vi "TLB Native Dynamic Events ver 0.05b queue mode.vi"() -> ()   [LabVIEW 2018]
uses:
  Labview Training Phase 2/Enum Controls/States for Action Engine.ctl
  Type def/TLB event states.ctl
  Type def/TLB MHL States.ctl
  <vilib>/Studica/Studica Toolkit/NavX/NavX.lvlib
  <vilib>/Studica/Studica Toolkit/Background/I2C Channel.ctl
  <vilib>/myRIO/Common/Instrument Driver Framework/myRIO v1.0/AI/typedefs/AI Channels Enum.ctl
  <vilib>/myRIO/Common/Instrument Driver Framework/myRIO v1.0/AI/typedefs/AI Channels List.ctl
panel:
  out "Sharp IR Distance 2":dbl
  out "Sharp IR Distance":dbl
  out "YRPHfH":T1
  out "Displacement":T2
  out "LinearAcceleration":T3
  out "NavX Info Out":T5
  out "Distance":T6
  out "Speed":T7
  in  "xTargetSpeed":dbl
  in  "yTargetSpeed":dbl
  in  "wTargetSpeed":dbl
  out "Action Queues":string[](array[string])
  out "State logic":T8
  out "Action State":string
  in  "Task condition":bool
  in  "Combo Box":string(combo)
  in  "Stop Queue":bool
  in  "Start Task":bool
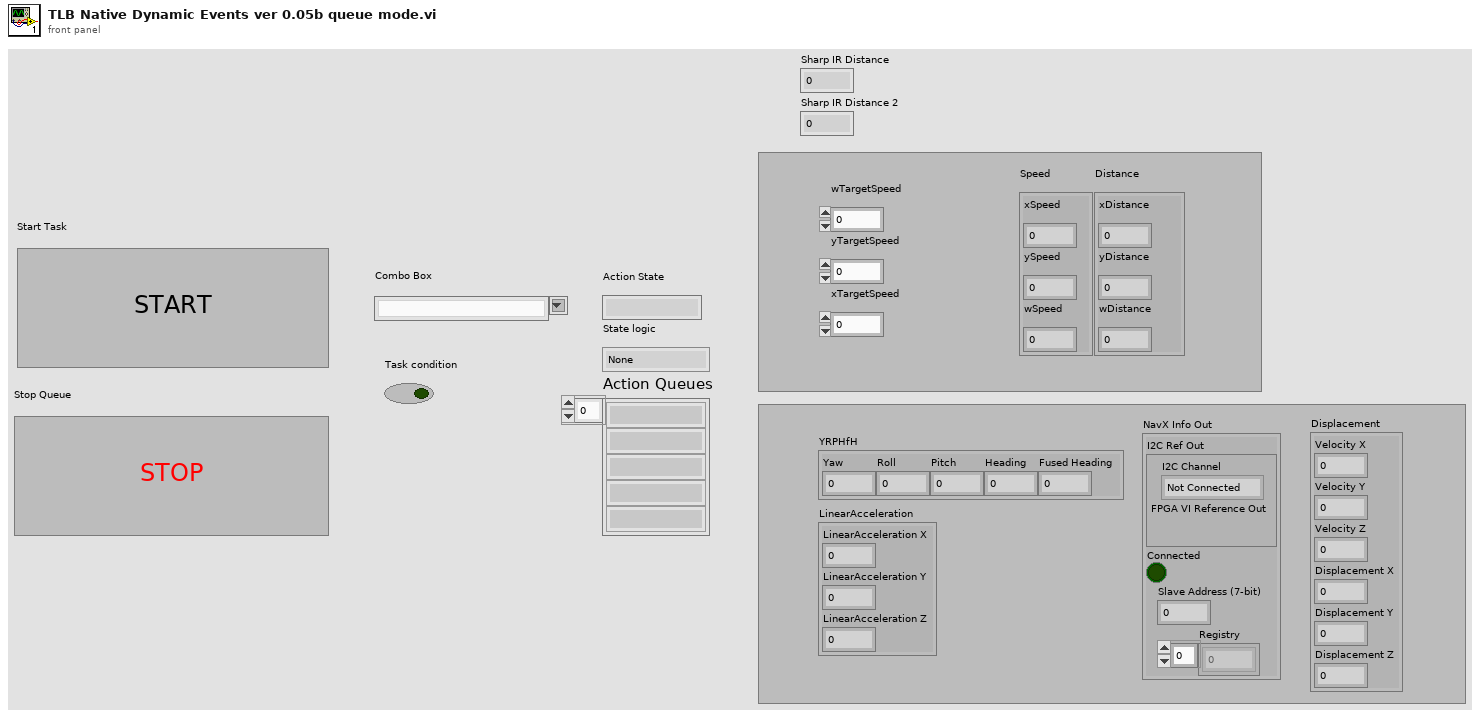
[diagram p1: front panel]
types:
  T1 = cluster{"Yaw":dbl, "Roll":dbl, "Pitch":dbl, "Heading":dbl, "Fused Heading":dbl}
  T2 = cluster{"Velocity X":dbl, "Velocity Y":dbl, "Velocity Z":dbl, "Displacement X":dbl, "Displacement Y":dbl, "Displacement Z":dbl}
  T3 = cluster{"LinearAcceleration X":dbl, "LinearAcceleration Y":dbl, "LinearAcceleration Z":dbl}
  T4 = typedef "I2C Channel.ctl" = enum16{"Not Connected", "A", "B"}
  T5 = cluster{"I2C Ref Out":cluster{"I2C Channel":T4, "FPGA VI Reference Out":refnum<k20>}, "Connected":bool, "Slave Address (7-bit)":u8, "Registry":u8[]}
  T6 = cluster{"xDistance":dbl, "yDistance":dbl, "wDistance":dbl}
  T7 = cluster{"xSpeed":dbl, "ySpeed":dbl, "wSpeed":dbl}
  T8 = typedef "TLB MHL States.ctl" = enum16{"None", "Startup", "Idle", "Processing", "Shutdown", "Reset", "Task 1", "Task 2", "Task 3", "Task 4", "Task 4a", "Task 4b", "Task 4c", "Task 4d", "Task 4e", "Task 4f", "Task 4g", "Task 4h", "Acquire image", "Wall follow mode", "Drive Straight"}
  T9 = typedef "States for Action Engine.ctl" = enum16{"Initialize", "Write", "Read"}
  T10 = typedef "TLB event states.ctl" = enum16{"Start Sequence", "Exit", "Start Task 1", "Start Task 2", "Start Task 3", "Start Task 4", "Camera vision", "Wall follow mode", "Idle", "Start Drive Straight"}
  T11 = typedef "TLB event states.ctl" = enum16{"Start Sequence", "Exit", "Task 1", "Task 2", "Idle"}
  T12 = cluster{"queue out":refnum<queue>, "error out":errorcluster}
  T13 = typedef "AI Channels List.ctl" = T14[]
  T14 = typedef "AI Channels Enum.ctl" = enum16{"Not Connected", "AudioIn/Left", "AudioIn/Right", "C/AI0", "C/AI1", "A/AI0", "A/AI1", "A/AI2", "A/AI3", "A/AI4", "A/AI5", "A/AI6", "A/AI7", "B/AI0", "B/AI1", "B/AI2", "B/AI3", "B/AI4", "B/AI5", "B/AI6", "B/AI7", "AI/AI0", "AI/AI1", "AI/AI2", "AI/AI3", "A/AI0 (DIFF)", "A/AI1 (DIFF)", "A/AI2 (DIFF)", "A/AI3 (DIFF)", "B/AI0 (DIFF)", "B/AI1 (DIFF)", "B/AI2 (DIFF)", "B/AI3 (DIFF)"}
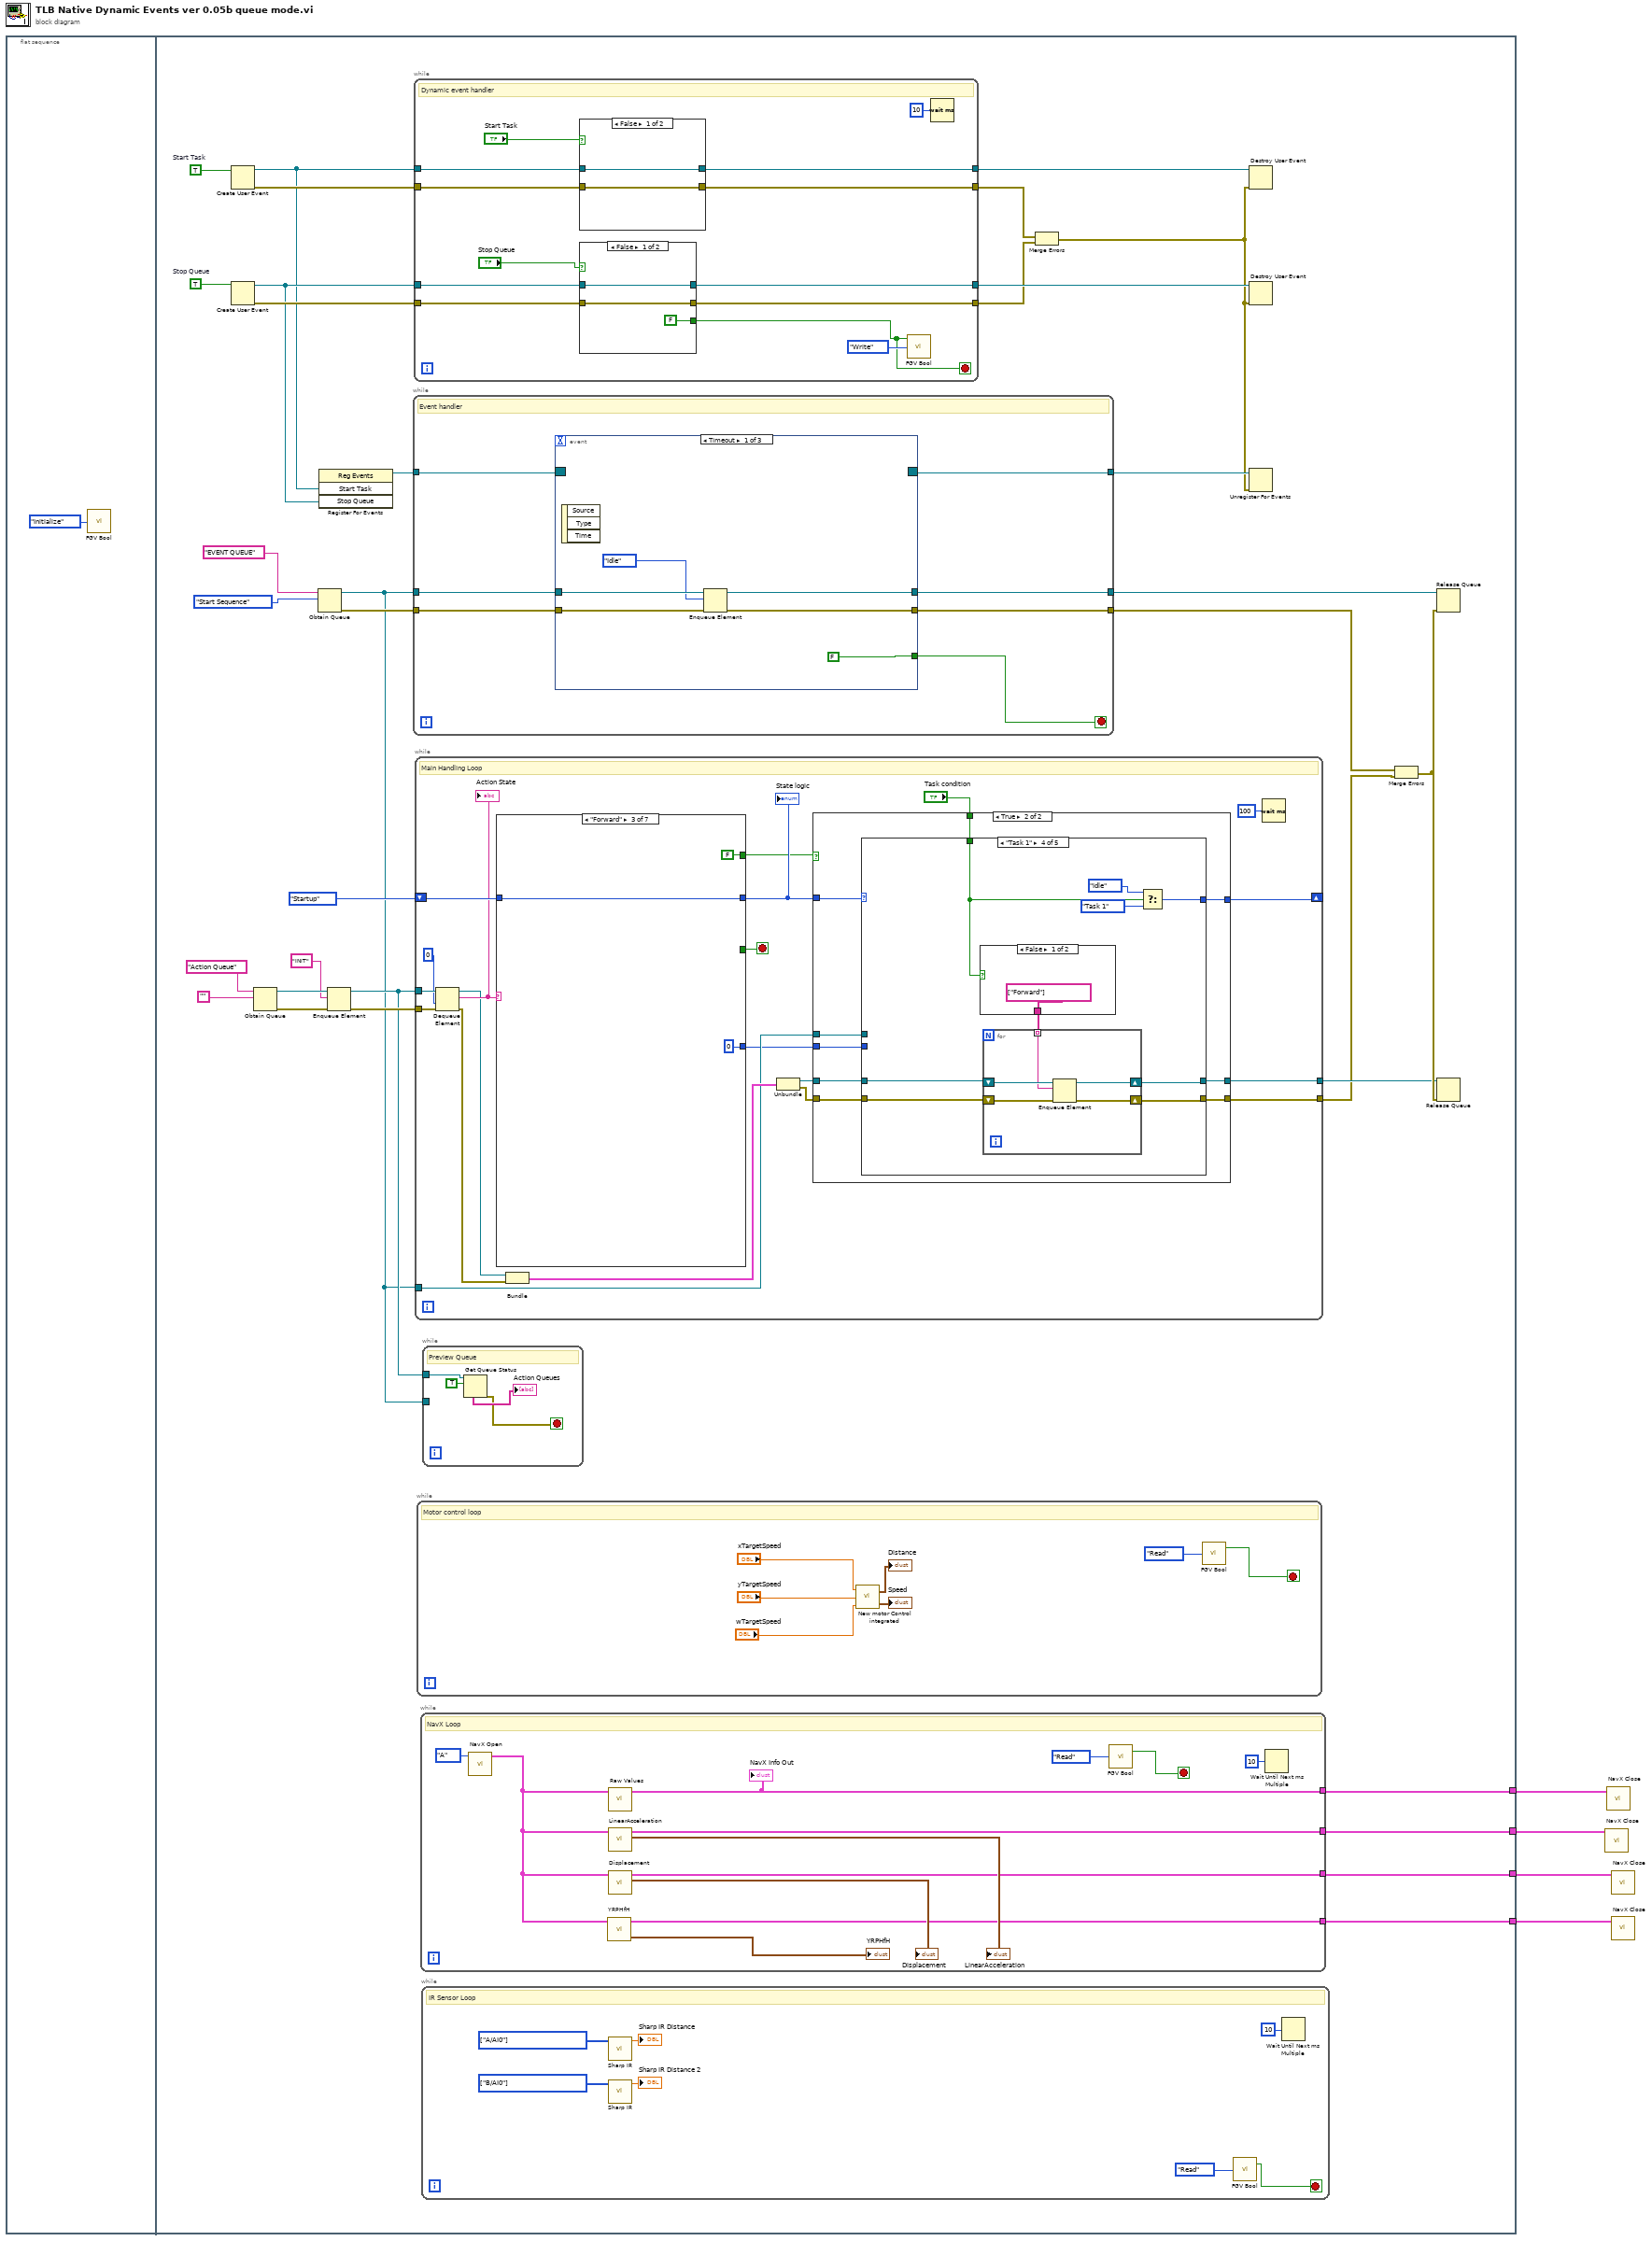
[diagram p0: block diagram]
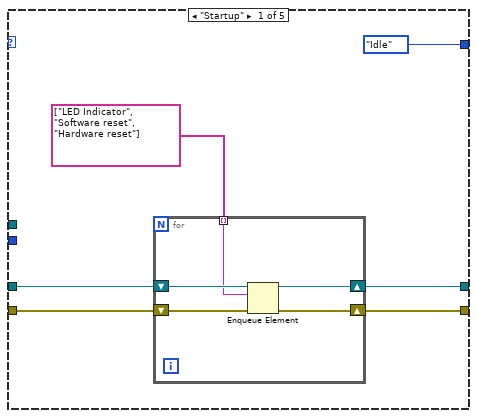
[diagram p3: hidden frame]
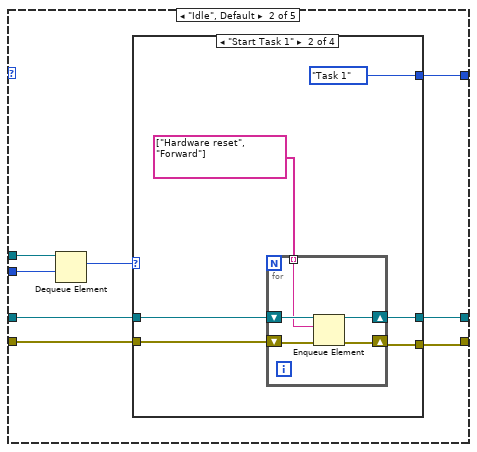
[diagram p4: hidden frame]
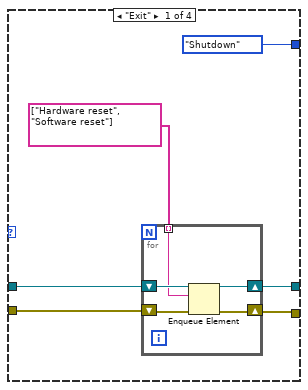
[diagram p5: hidden frame]
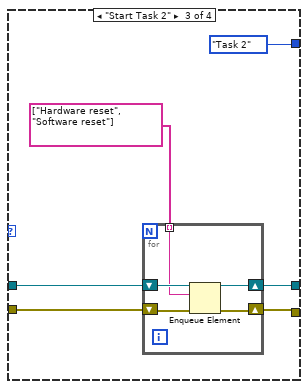
[diagram p6: hidden frame]
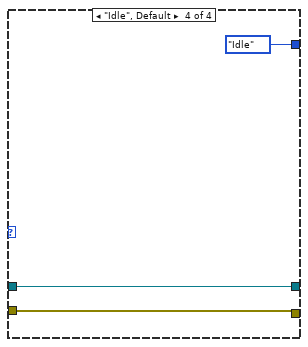
[diagram p7: hidden frame]
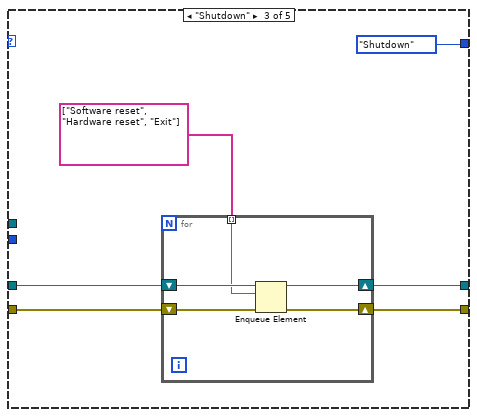
[diagram p8: hidden frame]
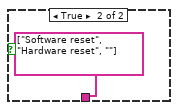
[diagram p9: hidden frame]
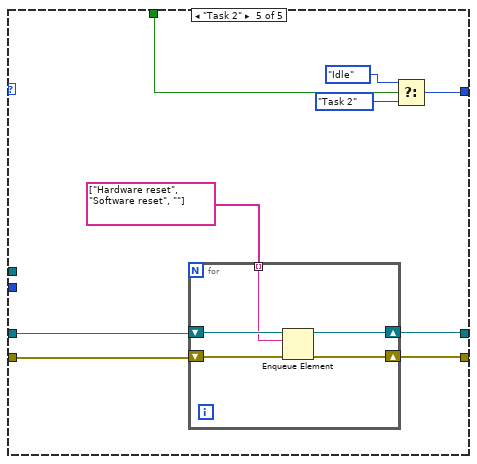
[diagram p10: hidden frame]
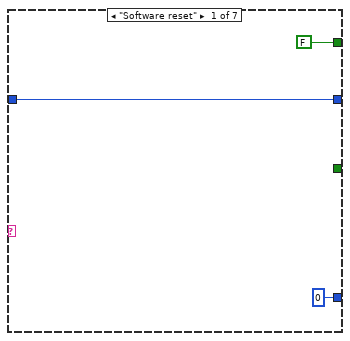
[diagram p11: hidden frame]
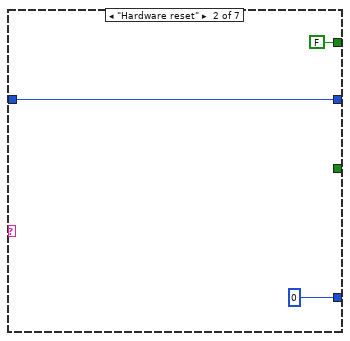
[diagram p12: hidden frame]
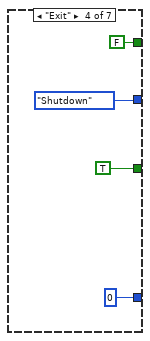
[diagram p13: hidden frame]
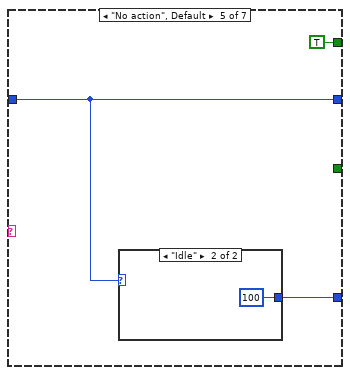
[diagram p14: hidden frame]
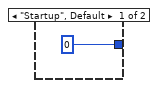
[diagram p15: hidden frame]
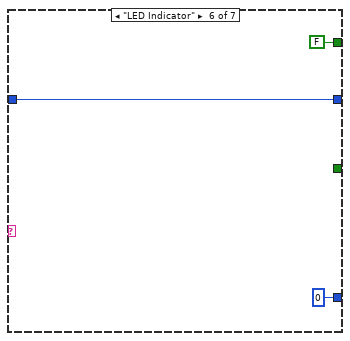
[diagram p16: hidden frame]
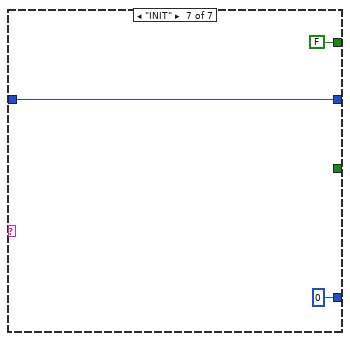
[diagram p17: hidden frame]
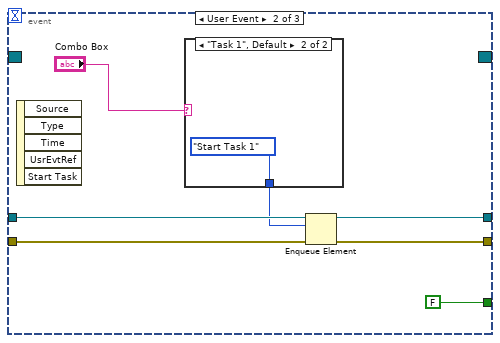
[diagram p18: hidden frame]
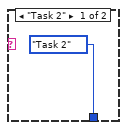
[diagram p19: hidden frame]
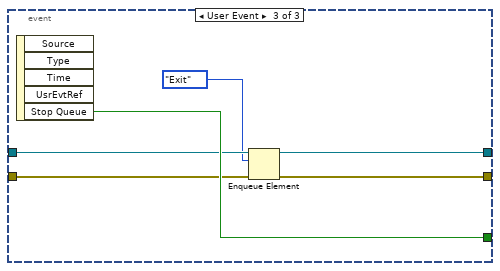
[diagram p20: hidden frame]
diagram:
  n1 = flat-sequence {
    tunnel: [w9] -> w4
    tunnel: [w8] -> w3
    tunnel: [w7] -> w2
    tunnel: [w6] -> w1
    frame #0 {
      n2 = call "FGV Bool.vi"("Init/Read/Write State"=States_for_Action_Engine."Initialize") -> ()  [unwired: 2 in, 2 out]
    }
    frame #1 {
      w39 = TRUE  # Stop Queue
      w38 = TRUE  # Start Task
      n3 = Create User Event(user event datatype=w38) -> (user event=w30:refnum<user-event>, error out=w35:errorcluster)  [unwired: 1 in]
      n4 = Create User Event(user event datatype=w39) -> (user event=w31:refnum<user-event>, error out=w34:errorcluster)  [unwired: 1 in]
      n5 = Obtain Queue(name (unnamed)="Action Queue", element data type="") -> (queue out=w23:refnum<queue>, error out=w19:errorcluster)  [unwired: 3 in, 1 out]
      n6 = Obtain Queue(name (unnamed)="EVENT QUEUE", element data type=TLB_event_states."Start Sequence" ("Enum")) -> (queue out=w10:refnum<queue>, error out=w20:errorcluster)  [unwired: 3 in, 1 out]
      n7 = register-events(w30, w31) -> (reference out=w29:refnum<event-registration>)  [unwired: 2 in, 1 out]
      n8 = Enqueue Element(queue=w23, element="INIT", error in (no error)=w19) -> (queue out=w11:refnum<queue>, error out=w18:errorcluster)  [unwired: 1 in, 1 out]
      n9 = while {
        tunnel: w29 -> [w228]
        tunnel: [w227] -> w28
        tunnel: w10 -> [w225]
        tunnel: [w224] -> w27
        tunnel: w20 -> [w223]
        tunnel: [w222] -> w17
        stop <- w226 stop-if-true
        # "Event handler"
        n10 = event shown="[0] Timeout" {
          selector: w228 -> [_ _ _]
          dyn-events: [_ _ _] -> w227
          timeout: _ -> [_ _ _]
          tunnel: [FALSE FALSE w249] -> w226
          tunnel: w225 -> [w233 w240 w247]
          tunnel: [w232 w239 w248] -> w224
          tunnel: w223 -> [w230 w236 w245]
          tunnel: [w229 w235 w244] -> w222
          event Timeout {
            n11 = event-data() -> ()  [unwired: 1 in, 3 out]
            n12 = Enqueue Element(queue=w233, element=TLB_event_states."Idle" ("Enum"), error in (no error)=w230) -> (queue out=w232:refnum<queue>, error out=w229:errorcluster)  [unwired: 1 in, 1 out]
          }
          event User Event {
            n13 = event-data() -> ()  [unwired: 1 in, 5 out]
            n14 = case shown="\"Task 1\", Default" "Combo Box" {
              tunnel: [TLB_event_states."Task 2" ("Enum") TLB_event_states."Start Task 1" ("Enum")] -> w237
              frame "Task 2" {
              }
              frame "Task 1", Default {
              }
            }
            n15 = Enqueue Element(queue=w240, element=w237, error in (no error)=w236) -> (queue out=w239:refnum<queue>, error out=w235:errorcluster)  [unwired: 1 in, 1 out]
          }
          event User Event {
            n16 = event-data() -> ("Stop Queue"=w249:bool)  [unwired: 1 in, 4 out]
            n17 = Enqueue Element(queue=w247, element=TLB_event_states."Exit" ("Enum"), error in (no error)=w245) -> (queue out=w248:refnum<queue>, error out=w244:errorcluster)  [unwired: 1 in, 1 out]
          }
        }
      }
      n18 = while {
        tunnel: w30 -> [w261]
        tunnel: w31 -> [w260]
        tunnel: [w259] -> w37
        tunnel: [w258] -> w36
        tunnel: w35 -> [w257]
        tunnel: [w256] -> w33
        tunnel: w34 -> [w255]
        tunnel: [w254] -> w32
        stop <- w250 stop-if-true
        # "Dynamic event handler"
        n19 = case shown="False" "Start Task" {
          selector: "Start Task" -> [_ w273]
          tunnel: w261 -> [w272 w277]
          tunnel: [w272 w276] -> w258
          tunnel: w257 -> [w271 w275]
          tunnel: [w271 w274] -> w256
          frame False {
          }
          frame True {
            n20 = Generate User Event(user event=w277, event data cluster=w273, error in=w275) -> (user event out=w276:refnum<user-event>, error out=w274:errorcluster)  [unwired: 1 in]
          }
        }
        n21 = case shown="False" "Stop Queue" {
          selector: "Stop Queue" -> [_ w266]
          tunnel: w260 -> [w265 w270]
          tunnel: [w265 w269] -> w259
          tunnel: w255 -> [w264 w268]
          tunnel: [w264 w267] -> w254
          tunnel: [FALSE w266] -> w250
          frame False {
          }
          frame True {
            n22 = Generate User Event(user event=w270, event data cluster=w266, error in=w268) -> (user event out=w269:refnum<user-event>, error out=w267:errorcluster)  [unwired: 1 in]
          }
        }
        n23 = call "FGV Bool.vi"("Init/Read/Write State"=States_for_Action_Engine."Write", "Input Node"=w250) -> ()  [unwired: 1 in, 2 out]
        n24 = Wait (ms)(milliseconds to wait=u32 10) -> ()  [unwired: 1 out]
      }
      n25 = while {
        tunnel: w10 -> [w75]
        shift-right: [w76] -> _
        shift-left: TLB_MHL_States."Startup" ("Enum") -> [w88]
        tunnel: w11 -> [w86]
        tunnel: w18 -> [w84]
        tunnel: [w78] -> w15
        tunnel: [w77] -> w14
        stop <- w73 stop-if-true
        # "Main Handling Loop"
        n26 = Dequeue Element(queue=w86, timeout in ms (-1)=0, error in (no error)=w84) -> (queue out=w83:refnum<queue>, element=w85:string, error out=w82:errorcluster)  [unwired: 1 out]
        "Action State" <- w85
        n27 = case shown="\"Forward\"" w85 {
          tunnel: [w200 w203 w205 TLB_MHL_States."Shutdown" ("Enum") w213 w218 w221] -> w87
          tunnel: w88 -> [w200 w203 w205 _ w213 w218 w221]
          tunnel: [0 0 0 0 w212 0 0] -> w74
          tunnel: [_ _ _ TRUE _ _ _] -> w73
          tunnel: [FALSE FALSE FALSE FALSE TRUE FALSE FALSE] -> w71
          frame "Software reset" {
          }
          frame "Hardware reset" {
          }
          frame "Forward" {
          }
          frame "Exit" {
          }
          frame "No action", Default {
            n28 = case shown="\"Idle\"" w213 {
              tunnel: [0 100] -> w212
              frame "Startup", Default {
              }
              frame "Idle" {
              }
            }
          }
          frame "LED Indicator" {
          }
          frame "INIT" {
          }
        }
        "State logic" <- w87
        n29 = Bundle("queue out"=w83, "error out"=w82) -> (w81:T12)  [unwired: 1 in]
        n30 = Unbundle(w81) -> ("queue out"=w80:refnum<queue>, "error out"=w79:errorcluster)
        n31 = case shown="True" w71 {
          tunnel: w87 -> [w91 w101]
          tunnel: w80 -> [w92 w100]
          tunnel: w79 -> [w90 w99]
          tunnel: [w92 w98] -> w78
          tunnel: [w90 w97] -> w77
          tunnel: [w91 w96] -> w76
          tunnel: w75 -> [_ w95]
          tunnel: w74 -> [_ w94]
          tunnel: "Task condition" -> [_ w93]
          frame False {
          }
          frame True {
            n32 = case shown="\"Task 1\"" w101 {
              tunnel: w100 -> [w107 w114 w160 w171 w186]
              tunnel: w99 -> [w106 w116 w158 w170 w185]
              tunnel: [w105 w117 w159 w173 w188] -> w98
              tunnel: [w104 w115 w157 w172 w187] -> w97
              tunnel: [TLB_MHL_States."Idle" ("Enum") w118 TLB_MHL_States."Shutdown" ("Enum") w174 w190] -> w96
              tunnel: w95 -> [_ w120 _ _ _]
              tunnel: w94 -> [_ w113 _ _ _]
              tunnel: w93 -> [_ _ _ w169 w184]
              frame "Startup" {
                n33 = for {
                  shift-right: [w110] -> w105
                  shift-left: w107 -> [w112]
                  shift-right: [w109] -> w104
                  shift-left: w106 -> [w111]
                  tunnel: string[] ["LED Indicator", "Software reset", "Hardware reset"] -> [w108] mode=indexing
                  n34 = Enqueue Element(queue=w112, element=w108, error in (no error)=w111) -> (queue out=w110:refnum<queue>, error out=w109:errorcluster)  [unwired: 1 in, 1 out]
                }
              }
              frame "Idle", Default {
                n35 = Dequeue Element(queue=w120, timeout in ms (-1)=w113) -> (element=w119:T10)  [unwired: 1 in, 3 out]
                n36 = case shown="\"Start Task 1\"" w119 {
                  tunnel: [TLB_MHL_States."Shutdown" ("Enum") TLB_MHL_States."Task 1" ("Enum") TLB_MHL_States."Task 2" ("Enum") TLB_MHL_States."Idle" ("Enum")] -> w118
                  tunnel: [w123 w136 w145 w155] -> w117
                  tunnel: w114 -> [w125 w135 w147 w155]
                  tunnel: w116 -> [w124 w134 w146 w154]
                  tunnel: [w122 w133 w144 w154] -> w115
                  frame "Exit" {
                    n37 = for {
                      shift-right: [w131] -> w123
                      shift-left: w125 -> [w130]
                      shift-right: [w128] -> w122
                      shift-left: w124 -> [w129]
                      tunnel: string[] ["Hardware reset", "Software reset"] -> [w127] mode=indexing
                      n38 = Enqueue Element(queue=w130, element=w127, error in (no error)=w129) -> (queue out=w131:refnum<queue>, error out=w128:errorcluster)  [unwired: 1 in, 1 out]
                    }
                  }
                  frame "Start Task 1" {
                    n39 = for {
                      shift-right: [w142] -> w136
                      shift-left: w135 -> [w141]
                      shift-right: [w139] -> w133
                      shift-left: w134 -> [w140]
                      tunnel: string[] ["Hardware reset", "Forward"] -> [w138] mode=indexing
                      n40 = Enqueue Element(queue=w141, element=w138, error in (no error)=w140) -> (queue out=w142:refnum<queue>, error out=w139:errorcluster)  [unwired: 1 in, 1 out]
                    }
                  }
                  frame "Start Task 2" {
                    n41 = for {
                      shift-right: [w153] -> w145
                      shift-left: w147 -> [w152]
                      shift-right: [w150] -> w144
                      shift-left: w146 -> [w151]
                      tunnel: string[] ["Hardware reset", "Software reset"] -> [w149] mode=indexing
                      n42 = Enqueue Element(queue=w152, element=w149, error in (no error)=w151) -> (queue out=w153:refnum<queue>, error out=w150:errorcluster)  [unwired: 1 in, 1 out]
                    }
                  }
                  frame "Idle", Default {
                  }
                }
              }
              frame "Shutdown" {
                n43 = for {
                  shift-right: [w165] -> w159
                  shift-left: w160 -> [w167]
                  shift-right: [w164] -> w157
                  shift-left: w158 -> [w166]
                  tunnel: string[] ["Software reset", "Hardware reset", "Exit"] -> [w163] mode=indexing
                  n44 = Enqueue Element(queue=w167, element=w163, error in (no error)=w166) -> (queue out=w165:refnum<queue>, error out=w164:errorcluster)  [unwired: 1 in, 1 out]
                }
              }
              frame "Task 1" {
                n45 = case shown="False" w169 {
                  tunnel: [string[] ["Forward"] string[] ["Software reset", "Hardware reset", ""]] -> w168
                  frame False {
                  }
                  frame True {
                  }
                }
                n46 = for {
                  shift-right: [w181] -> w173
                  shift-left: w171 -> [w183]
                  shift-right: [w180] -> w172
                  shift-left: w170 -> [w182]
                  tunnel: w168 -> [w179] mode=indexing
                  n47 = Enqueue Element(queue=w183, element=w179, error in (no error)=w182) -> (queue out=w181:refnum<queue>, error out=w180:errorcluster)  [unwired: 1 in, 1 out]
                }
                n48 = Select(t=TLB_MHL_States."Idle" ("Enum"), s=w169, f=TLB_MHL_States."Task 1" ("Enum")) -> (s? t:f=w174:T8)
              }
              frame "Task 2" {
                n49 = for {
                  shift-right: [w195] -> w188
                  shift-left: w186 -> [w197]
                  shift-right: [w194] -> w187
                  shift-left: w185 -> [w196]
                  tunnel: string[] ["Hardware reset", "Software reset", ""] -> [w193] mode=indexing
                  n50 = Enqueue Element(queue=w197, element=w193, error in (no error)=w196) -> (queue out=w195:refnum<queue>, error out=w194:errorcluster)  [unwired: 1 in, 1 out]
                }
                n51 = Select(t=TLB_MHL_States."Idle" ("Enum"), s=w184, f=TLB_MHL_States."Task 2" ("Enum")) -> (s? t:f=w190:T8)
              }
            }
          }
        }
        n52 = Wait (ms)(milliseconds to wait=u32 100) -> ()  [unwired: 1 out]
      }
      n53 = while {
        stop <- w64 stop-if-true
        # "Motor control loop"
        n54 = call "New motor Control integrated.vi"("wTargetSpeed"="wTargetSpeed", "yTargetSpeed"="yTargetSpeed", "xTargetSpeed"="xTargetSpeed") -> ("Speed"=→"Speed":T7, "Distance"=→"Distance":T6)
        n55 = call "FGV Bool.vi"("Init/Read/Write State"=States_for_Action_Engine."Read") -> ("Output node"=w64:bool)  [unwired: 2 in, 1 out]
      }
      n56 = while {
        tunnel: [w55] -> w9
        tunnel: [w51] -> w8
        tunnel: [w50] -> w7
        tunnel: [w49] -> w6
        stop <- w57 stop-if-true
        # "NavX Loop"
        n57 = call <vilib>:"NavX Open.vi"("I2C Channel"=I2C_Channel."A") -> ("NavX Info"=w47:T5)  [unwired: 9 in, 1 out]
        n58 = call <vilib>:"YRPHfH.vi"("NavX Info In"=w47) -> ("YRPHfH"=→"YRPHfH":T1, "NavX Info Out"=w50:T5)  [unwired: 3 in]
        n59 = call <vilib>:"Raw Values.vi"("NavX Info In"=w47) -> ("NavX Info Out"=w55:T5)  [unwired: 8 in, 1 out]
        "NavX Info Out" <- w55
        n60 = call <vilib>:"LinearAcceleration.vi"("NavX Info In"=w47) -> ("LinearAcceleration"=→"LinearAcceleration":T3, "NavX Info Out"=w51:T5)  [unwired: 9 in]
        n61 = call <vilib>:"Displacement.vi"("NavX Info In"=w47) -> ("Displacement"=→"Displacement":T2, "NavX Info Out"=w49:T5)  [unwired: 9 in]
        n62 = call "FGV Bool.vi"("Init/Read/Write State"=States_for_Action_Engine."Read") -> ("Output node"=w57:bool)  [unwired: 2 in, 1 out]
        n63 = Wait Until Next ms Multiple(millisecond multiple=u32 10) -> ()  [unwired: 1 out]
      }
      n64 = while {
        stop <- w40 stop-if-true
        w45 = T13 [enum."B/AI0"] items=["Not Connected", "AudioIn/Left", "AudioIn/Right", "C/AI0", "C/AI1", "A/AI0", "A/AI1", "A/AI2", "A/AI3", "A/AI4", "A/AI5", "A/AI6", "A/AI7", "B/AI0", "B/AI1", "B/AI2", "B/AI3", "B/AI4", "B/AI5", "B/AI6", "B/AI7", "AI/AI0", "AI/AI1", "AI/AI2", "AI/AI3", "A/AI0 (DIFF)", "A/AI1 (DIFF)", "A/AI2 (DIFF)", "A/AI3 (DIFF)", "B/AI0 (DIFF)", "B/AI1 (DIFF)", "B/AI2 (DIFF)", "B/AI3 (DIFF)"] ("AI Channel")
        w46 = T13 [enum."A/AI0"] items=["Not Connected", "AudioIn/Left", "AudioIn/Right", "C/AI0", "C/AI1", "A/AI0", "A/AI1", "A/AI2", "A/AI3", "A/AI4", "A/AI5", "A/AI6", "A/AI7", "B/AI0", "B/AI1", "B/AI2", "B/AI3", "B/AI4", "B/AI5", "B/AI6", "B/AI7", "AI/AI0", "AI/AI1", "AI/AI2", "AI/AI3", "A/AI0 (DIFF)", "A/AI1 (DIFF)", "A/AI2 (DIFF)", "A/AI3 (DIFF)", "B/AI0 (DIFF)", "B/AI1 (DIFF)", "B/AI2 (DIFF)", "B/AI3 (DIFF)"] ("AI Channel")
        # "IR Sensor Loop"
        n65 = call <vilib>:"Sharp IR.vi"("AI Channel"=w46) -> ("Sharp IR Distance"=→"Sharp IR Distance":dbl)  [unwired: 8 in, 2 out]
        n66 = call <vilib>:"Sharp IR.vi"("AI Channel"=w45) -> ("Sharp IR Distance"=→"Sharp IR Distance 2":dbl)  [unwired: 8 in, 2 out]
        n67 = call "FGV Bool.vi"("Init/Read/Write State"=States_for_Action_Engine."Read") -> ("Output node"=w40:bool)  [unwired: 2 in, 1 out]
        n68 = Wait Until Next ms Multiple(millisecond multiple=u32 10) -> ()  [unwired: 1 out]
      }
      n69 = while {
        tunnel: w11 -> [w67]
        tunnel: w10 -> [_]
        stop <- w66 stop-if-true
        # "Preview Queue"
        n70 = Get Queue Status(queue=w67, return elements? (F)=TRUE) -> (error out=w66:errorcluster, elements=→"Action Queues":string[])  [unwired: 1 in, 6 out]
      }
      n71 = Merge Errors(w33, w32) -> (w13:errorcluster)
      n72 = Destroy User Event(user event=w36, error in=w13) -> ()  [unwired: 1 out]
      n73 = Destroy User Event(user event=w37, error in=w13) -> ()  [unwired: 1 out]
      n74 = Unregister For Events(event registration refnum=w28, error in=w13) -> ()  [unwired: 1 out]
      n75 = Merge Errors(w17, w14) -> (w16:errorcluster)
      n76 = Release Queue(queue=w27, error in (no error)=w16) -> ()  [unwired: 1 in, 3 out]
      n77 = Release Queue(queue=w15, error in (no error)=w16) -> ()  [unwired: 1 in, 3 out]
    }
  }
  n78 = call <vilib>:"NavX Close.vi"("NavX Info In"=w3) -> ()  [unwired: 10 in, 1 out]
  n79 = call <vilib>:"NavX Close.vi"("NavX Info In"=w4) -> ()  [unwired: 10 in, 1 out]
  n80 = call <vilib>:"NavX Close.vi"("NavX Info In"=w1) -> ()  [unwired: 10 in, 1 out]
  n81 = call <vilib>:"NavX Close.vi"("NavX Info In"=w2) -> ()  [unwired: 10 in, 1 out]
